vi "Destroy_Tag.vi"(8 "error in (no error)":errorcluster, 10 "Delete Children? (F)":bool, 11 "Tag_LVOOP in":refnum<class "Tree Tag Class.lvclass">) -> (0 "error out":errorcluster)   [LabVIEW 2012, in "Tree Tools.lvlib" / "Tree Tag Class.lvclass"]
uses:
  Tree Tag Class.lvclass
  Tree Tag Class.lvclass/Tree Tag Class.ctl
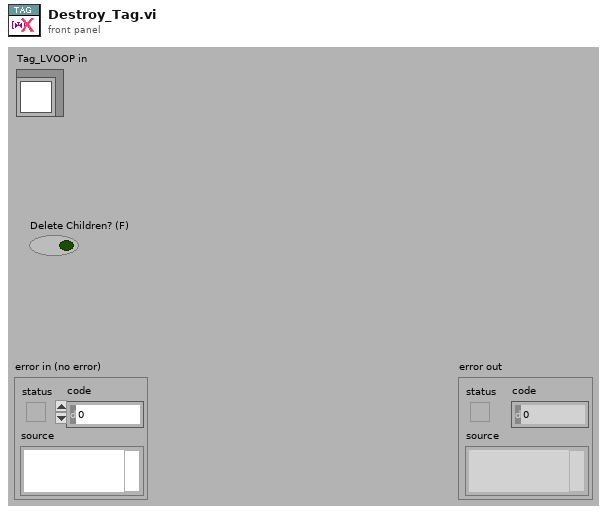
[diagram p1: front panel]
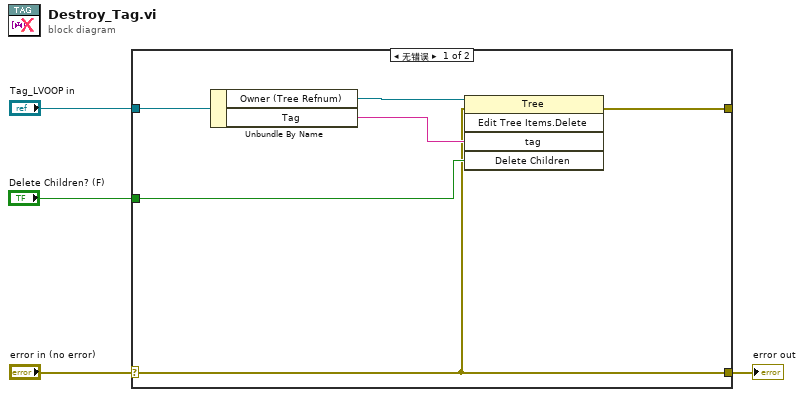
[diagram p0: block diagram]
diagram:
  n1 = case shown="无错误" "error in (no error)" {
    selector: "error in (no error)" -> [w5 w11]
    tunnel: [w5 w11] -> w3
    tunnel: "Tag_LVOOP in" -> [w10 _]
    tunnel: "Delete Children? (F)" -> [w7 _]
    tunnel: [w6 _] -> _
    frame No Error {
      n2 = Unbundle By Name(w10) -> ("Owner (Tree Refnum)"=w9:refnum<vi>, "Tag"=w8:string)
      n3 = invoke class="Tree" method="Edit Tree Items.Delete"(reference=w9, error in=w5, "tag"=w8, "Delete Children"=w7) -> (error out=w6:errorcluster)  [unwired: 1 in, 4 out]
    }
    frame Error {
    }
  }
  "error out" <- w3
